vi "Vision Research Phantom Series PhCon PhGetExactFrameRate.vi"(0 "CamVer":u32, 1 "SyncMode":T1, 2 "RequestedFrameRate":u32, 5 "Error In (no error)":errorcluster) -> (17 "pExactFrameRate":dbl, 19 "Error Out":errorcluster)   [LabVIEW 2013, in "VRI.lvlib"]
doc: "PhCon.dll\n\nPhGetExactFrameRate\nHRESULT PhGetExactFrameRate(UINT CamVer, UINT SyncMode, UINT RequestedFrameRate, \ndouble *pExactFrameRate)\n\nParameters Description\nCamVer (in) Camera version.\nSyncMode (in) Same value as SyncImaging field in the current aquisition \n parameters.\nRequestedFrameRate (in) Requested frame rate.\npExactFrameRate (out) The result: the exact frame rate this camera can realize, close to \n the requested one.\nReturn HRESULT (0 = Ok)\nComments Given a requested frame rate, this function computes the exact \n frame rate this camera is able to accomplish. The period \n corresponding to this frame rate has to be an exact multiple of\n the period of an internal clock: 250ns at the current Ethernet \n cameras.\n This routine does not check the result rate to be in the interval \n Min - Max. Call PhGetFrameRateRange() to check that."
uses:
  VRI.lvlib
  _Type Defs/PhCon SyncImaging.ctl
  Phantom DLLs/PhCon.Dll
panel:
  # "For instructions on the use of this VI, press Ctrl+H to display the help window and move the mouse over the icon, controls, and indicators"
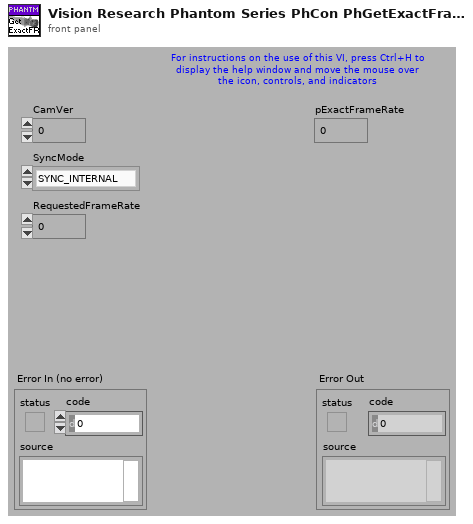
[diagram p1: front panel]
types:
  T1 = typedef "VRI.lvlib/PhCon SyncImaging.ctl" = enum32{"SYNC_INTERNAL", "SYNC_EXTERNAL", "SYNC_LOCKTOIRIG"}
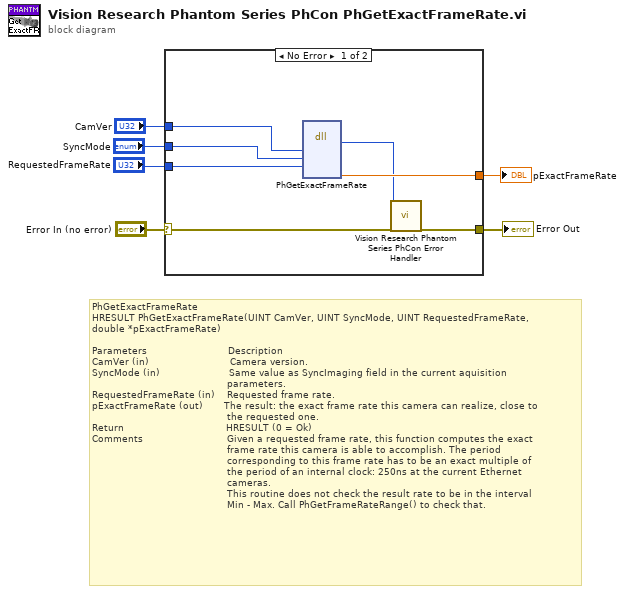
[diagram p0: block diagram]
diagram:
  # "PhGetExactFrameRate\nHRESULT PhGetExactFrameRate(UINT CamVer, UINT SyncMode, UINT RequestedFrameRate, \ndouble *pExactFrameRate)\n\nParameters                           Description\nCamVer (in)                           Camera version.\nSyncMode (in)                       Same value as SyncImaging field in the current aquisition \n                                             parameters.\nRequestedFrameRate (in)    Requested frame rate.\npExactFrameRate (out)       The result: the exact frame rate this camera can realize, close to \n                                             the requested one.\nReturn                                  HRESULT (0 = Ok)\nComments                            Given a requested frame rate, this function computes the exact \n                                             frame rate this camera is able to accomplish. The period \n                                             corresponding to this frame rate has to be an exact multiple of\n                                             the period of an internal clock: 250ns at the current Ethernet \n                                             cameras.\n                                             This routine does not check the result rate to be in the interval \n                                             Min - Max. Call PhGetFrameRateRange() to check that."
  n1 = case shown="No Error" "Error In (no error)" {
    selector: "Error In (no error)" -> [w13 w14]
    tunnel: [w12 w14] -> w5
    tunnel: "CamVer" -> [w11 _]
    tunnel: "SyncMode" -> [w10 _]
    tunnel: "RequestedFrameRate" -> [w9 _]
    tunnel: [w8 _] -> w1
    frame No Error {
      n2 = dll-call lib="C:/Projects/SDK/64-bit/Vision Research Phantom Series Labview Driver/Phantom DLLs/PhCon.dll" fn="PhGetExactFrameRate"("CamVer"=w11, "SyncMode"=w10, "RequestedFrameRate"=w9) -> ("HRESULT"=w7:i32, "pExactFrameRate"=w8:dbl)  [unwired: 5 in, 4 out]
      n3 = call "Vision Research Phantom Series PhCon Error Handler.vi"("ErrNo"=w7, "Error In (no error)"=w13) -> ("Error Out"=w12:errorcluster)  [unwired: 17 out]
    }
    frame Error {
    }
  }
  "Error Out" <- w5
  "pExactFrameRate" <- w1
